vi "SubtractZeroes.vi"(10 "RawPressure":dbl[][](array[numeric]), 11 "Zeroes":dbl[](array[numeric])) -> (3 "ZeroedPressure":dbl[][](array[numeric]))   [LabVIEW 2021]
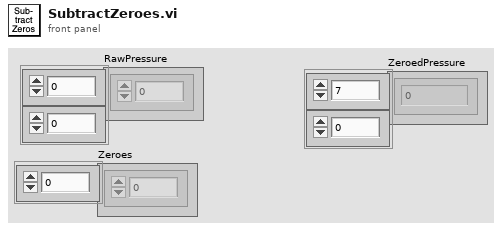
[diagram p1: front panel]
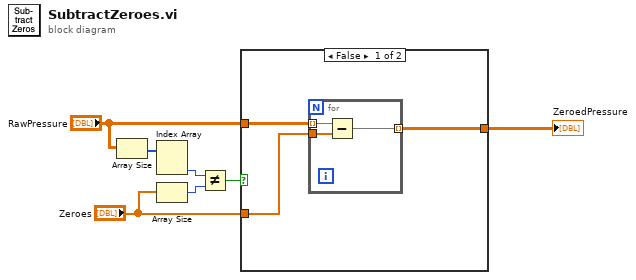
[diagram p0: block diagram]
diagram:
  n1 = Array Size(array="RawPressure") -> (size(s)=w5:i32[])
  n2 = Index Array(array=w5) -> (element #2=w3:i32)  [unwired: 2 in, 1 out]
  n3 = Array Size(array="Zeroes") -> (size(s)=w2:i32)
  n4 = Not Equal?(x=w3, y=w2) -> (x != y?=w1:bool)
  n5 = case shown="False" w1 {
    tunnel: "RawPressure" -> [w10 w14]
    tunnel: "Zeroes" -> [w9 _]
    tunnel: [w8 w14] -> w7
    frame False {
      n6 = for {
        tunnel: [w11] -> w8 mode=indexing
        tunnel: w10 -> [w13] mode=indexing
        tunnel: w9 -> [w12]
        n7 = Subtract(x=w13, y=w12) -> (x-y=w11:dbl[])
      }
    }
    frame True {
    }
  }
  "ZeroedPressure" <- w7
